vi "from table to pwm config.vi"(9 "PWM DC Index":i32[](array[numeric]), 10 "PWM Freq Index":i32[](array[numeric]), 11 "data table in":T1) -> (2 "PWM Config Array Out":cluster{"duty cycle":dbl, "frequency":dbl}[](array[cluster]), 3 "data table out":T1)   [LabVIEW 2015, in "DAQmx Module Runtime.lvclass"]
uses:
  DAQmx Module Runtime.lvclass
  <vilib>/NI/Tag Bus/table/data table.ctl
  <vilib>/NI/Tag Bus/table/data polymorphs/read many/read Doubles.vi
  <vilib>/NI/Tag Bus/table/data table.lvlib
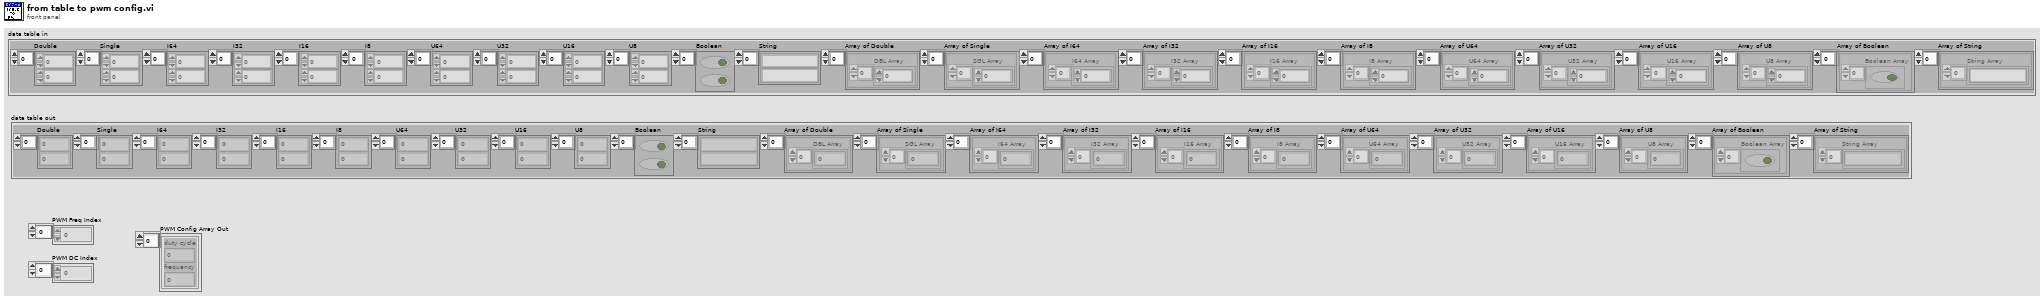
[diagram p1: front panel]
types:
  T1 = typedef "tag bus.lvlib/data table.lvlib/data table.ctl" = cluster{"Double":dbl[], "Single":sgl[], "I64":i64[], "I32":i32[], "I16":i16[], "I8":i8[], "U64":u64[], "U32":u32[], "U16":u16[], "U8":u8[], "Boolean":bool[], "String":string[], "Array of Double":cluster{"DBL Array":dbl[]}[], "Array of Single":cluster{"SGL Array":sgl[]}[], "Array of I64":cluster{"I64 Array":i64[]}[], "Array of I32":cluster{"I32 Array":i32[]}[], "Array of I16":cluster{"I16 Array":i16[]}[], "Array of I8":cluster{"I8 Array":i8[]}[], "Array of U64":cluster{"U64 Array":u64[]}[], "Array of U32":cluster{"U32 Array":u32[]}[], "Array of U16":cluster{"U16 Array":u16[]}[], "Array of U8":cluster{"U8 Array":u8[]}[], "Array of Boolean":cluster{"Boolean Array":bool[]}[], "Array of String":cluster{"String Array":string[]}[]}
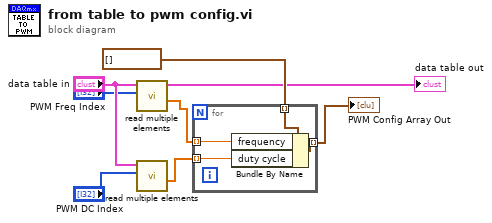
[diagram p0: block diagram]
diagram:
  n1 = call-poly <vilib>:"read multiple elements.vi"("indices"="PWM Freq Index", "data table in"="data table in") -> ("values"=w7:dbl[], "data table out"=→"data table out":T1)  [unwired: 8 in]
  n2 = call-poly <vilib>:"read multiple elements.vi"("indices"="PWM DC Index", "data table in"="data table in") -> ("values"=w8:dbl[])  [unwired: 8 in, 1 out]
  n3 = for {
    tunnel: cluster{"duty cycle":dbl, "frequency":dbl}[] [] ("data") -> [w12] mode=indexing
    tunnel: [w11] -> w6 mode=indexing
    tunnel: w7 -> [w10] mode=indexing
    tunnel: w8 -> [w9] mode=indexing
    n4 = Bundle By Name(cluster=w12, "frequency"=w10, "duty cycle"=w9) -> (w11:cluster{"duty cycle":dbl, "frequency":dbl})
  }
  "PWM Config Array Out" <- w6
